vi "Coords2Pixels.vi"(10 "Latitude":ext, 11 "Longitude":ext) -> (2 "Y":ext, 3 "X":ext)   [LabVIEW 2010]
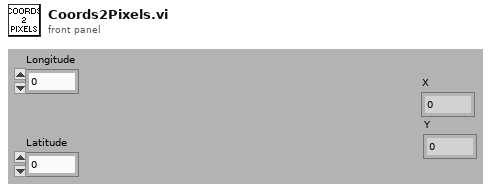
[diagram p1: front panel]
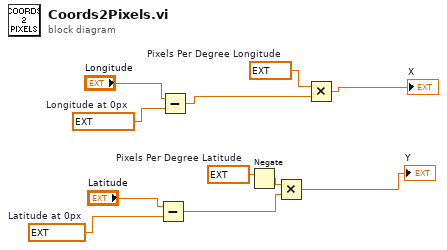
[diagram p0: block diagram]
diagram:
  w4 = ext 42.293996  # Latitude at 0px
  w5 = ext -71.264900999999999998  # Longitude at 0px
  w2 = ext 498829.0  # Pixels Per Degree Latitude
  w3 = ext 376430.0  # Pixels Per Degree Longitude
  n1 = Subtract(x="Latitude", y=w4) -> (x-y=w10:ext)
  n2 = Subtract(x="Longitude", y=w5) -> (x-y=w7:ext)
  n3 = Negate(x=w2) -> (-x=w1:ext)
  n4 = Multiply(x=w1, y=w10) -> (x*y=→"Y":ext)
  n5 = Multiply(x=w3, y=w7) -> (x*y=→"X":ext)
